vi "main.vi"   [LabVIEW 2016]
uses:
  MGCC_opal_RT/Communication (Montie Smith)/Initial Comm Test/Comm-BESS/DNP3_Master_Station_OpalRT.lvlib
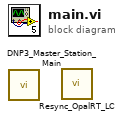
[diagram p0: block diagram]
diagram:
  n1 = call "DNP3_Master_Station_Main.vi"() -> ()  [unwired: 12 in]
  n2 = call "Resync_OpalRT_LC.vi"() -> ()  [unwired: 12 in]
